vi "EVM_Sweep_Only_R_S_CMP180_DebugMode.vi"() -> ()   [LabVIEW 2023, in "EVM.lvlib"]
uses:
  lib/CTL/LitePoint_EVM_SG.ctl
  lib/CTL/LitePoint_EVM_SA.ctl
  lib/CTL/JIO_FPGA_FTDI.ctl
  EVM.lvlib
  lib/LitePoints/LitePoints.lvlib
  lib/FTDI/JIO/CLC_JIO_FTDI.lvlib
  lib/R_S/R_S.lvlib
panel:
  in  "Init Func.":enum16{"ALL", "BFIC", "UDIC", "OFF"}(ring)
  in  "Recoder?":bool
  out "ReceivedPower":dbl format="%#.3g"
  out "Best EVM ALL":dbl
  out "PST(sec)":dbl
  out "Best EVM":dbl
  out "error out":errorcluster
  in  "Power res":i32=2
  in  "Stop Power":i32
  in  "Start Power":i32=-40
  in  "BFIC_ele_stop":i32=12
  in  "BFIC_ele_res":i32=4
  in  "BFIC_ele_start":i32
  in  "BFIC_com_stop":i32=12
  in  "BFIC_com_res":i32=4
  in  "BFIC_com_start":i32
  in  "UD_att_stop":i32=120
  in  "UD_att_res":i32=8
  in  "UD_att_start":i32
  out "UD_att":i32=255
  out "BFIC_com_step":i32=15
  out "BFIC_ele_step":i32=15
  out "SG Power":i32=-10
  in  "TRXmode":u16(ring)=1 items=["Tx"=1, "Rx"=2]
  in  "Polarity":u16(ring) items=["H", "V"]
  out "floder Exist?":bool=TRUE
  in  "Waiting \nTime(ms)":u32=1
  in  "FileNote":string="test16_wayne_MCS11"
  in  "SG":refnum<visa-resource-name>="TCPIP0::192.168.200.50::hislip0::INSTR"
  in  "SA":refnum<visa-resource-name>="TCPIP0::192.168.200.50::hislip0::INSTR"
  out "Spectrum Data":cluster{"X":dbl, "Y":dbl}[](graph)
  # "TMYTEK_CLC_JIO_R&S_EVM_CMP180_debugMode"
  # "12"
  # "12"
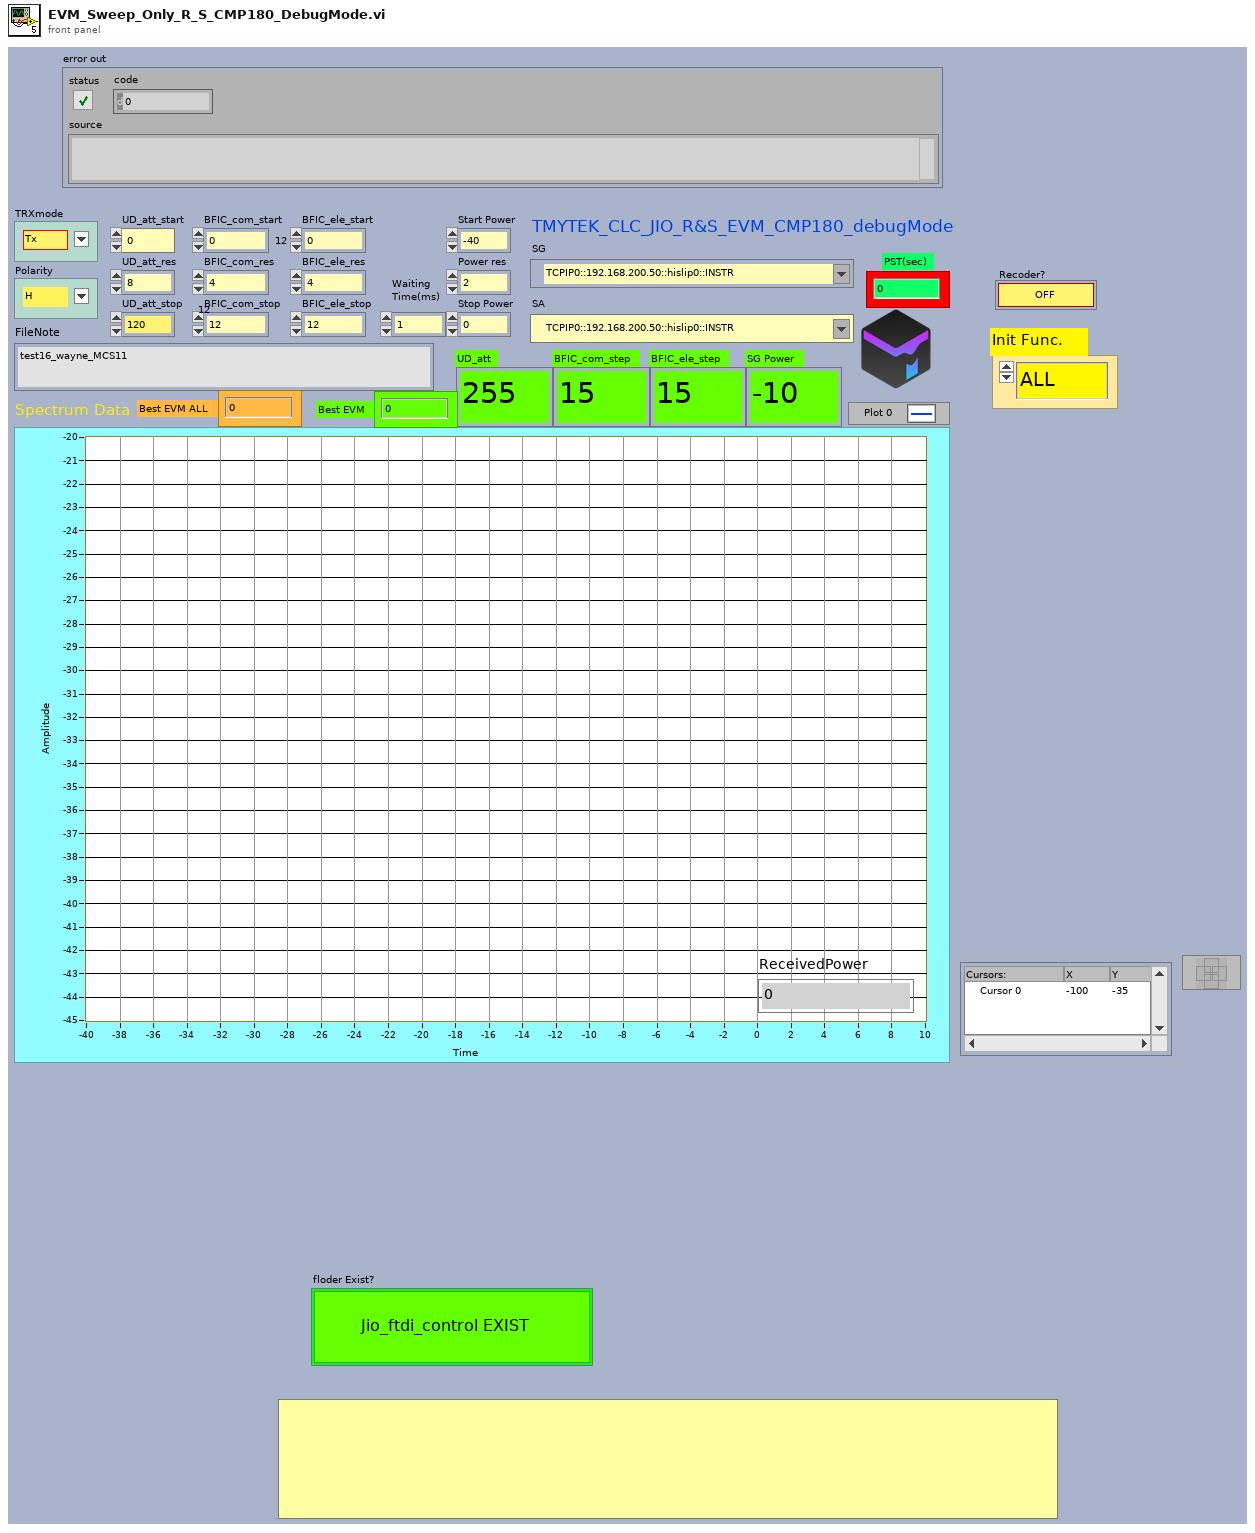
[diagram p1: front panel]
types:
  T1 = typedef "LitePoint_EVM_SG.ctl" = enum16{"Init", "Close", "set_SG", "AdjustLevel", "byPass", "RF_ON", "RF_OFF"}
  T2 = typedef "LitePoint_EVM_SA.ctl" = enum16{"Init", "Close", "set_SA", "get_EVM", "byPass", "getPower"}
  T3 = typedef "JIO_FPGA_FTDI.ctl" = enum16{"Init", "Close", "UD", "BFIC"}
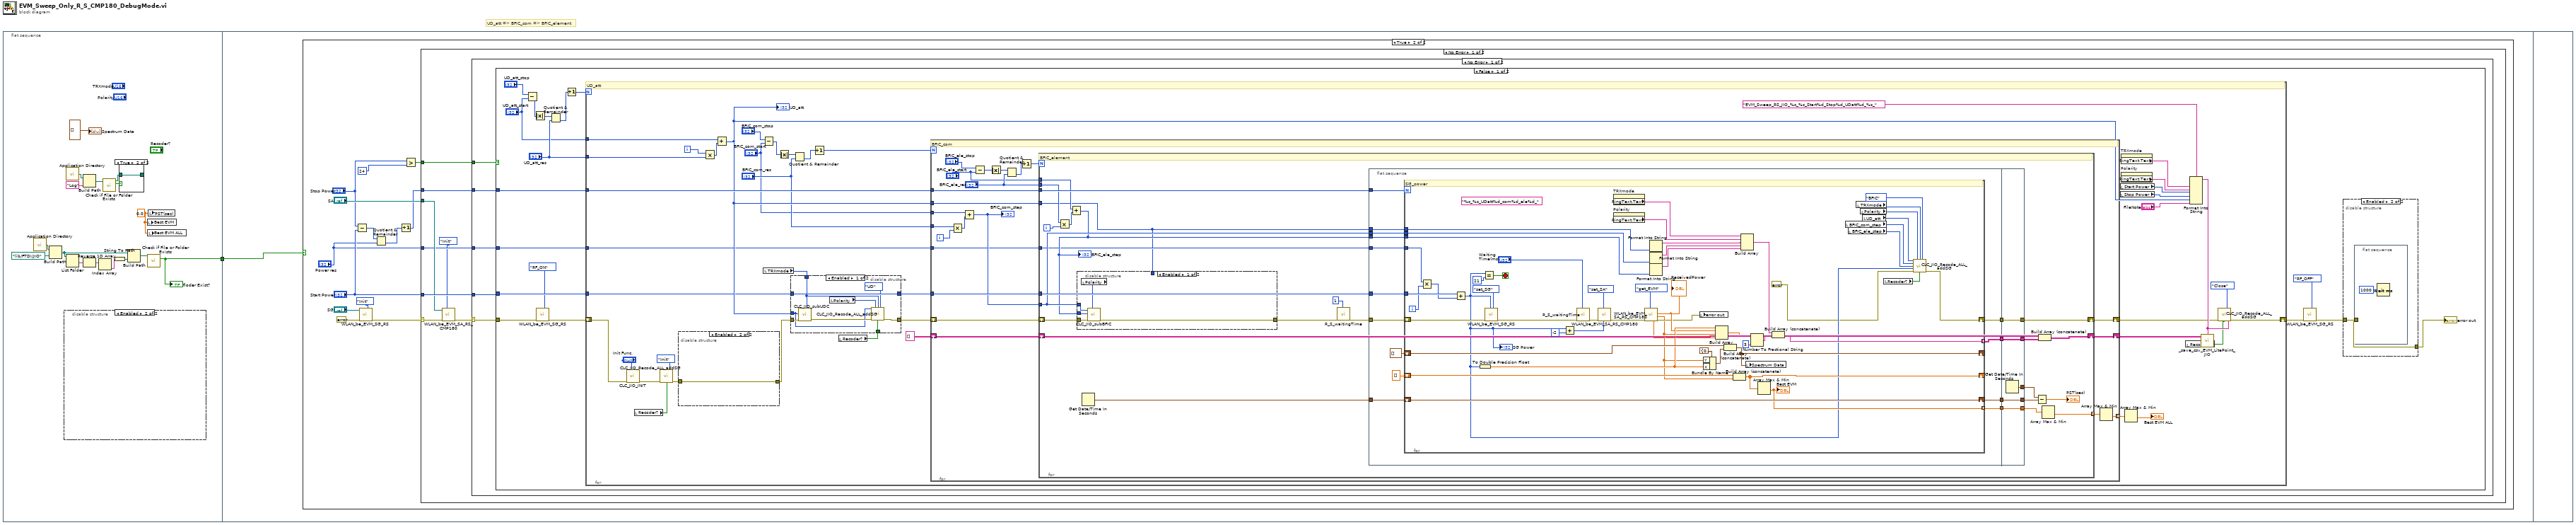
[diagram p0: block diagram]
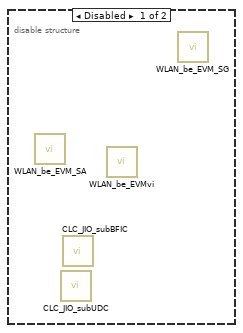
[diagram p2: hidden frame]
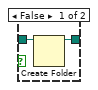
[diagram p3: hidden frame]
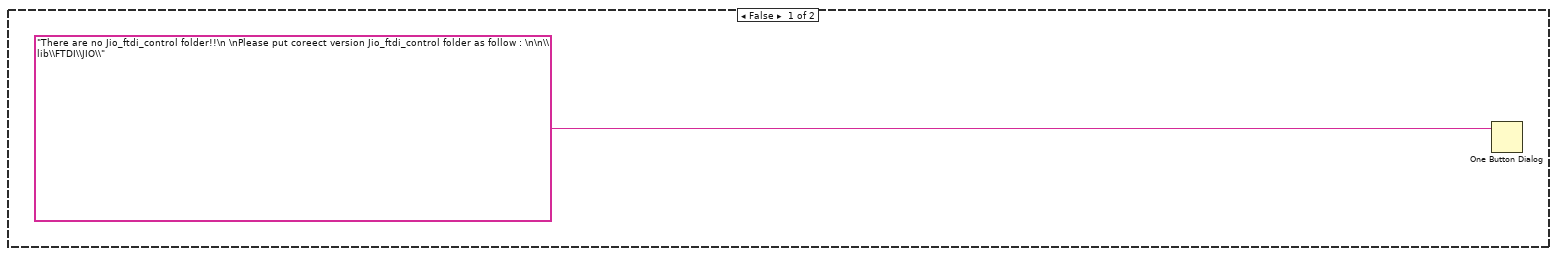
[diagram p4: hidden frame]
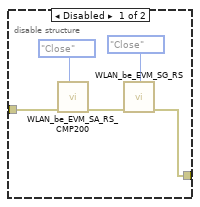
[diagram p5: hidden frame]
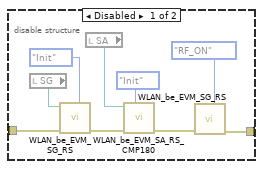
[diagram p6: hidden frame]
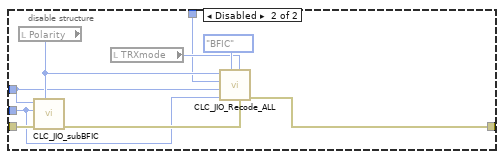
[diagram p8: hidden frame]
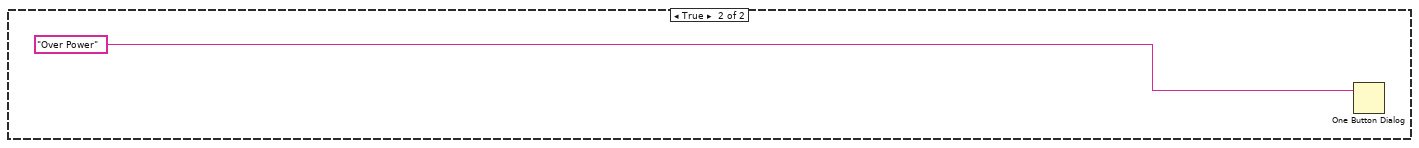
[diagram p9: hidden frame]
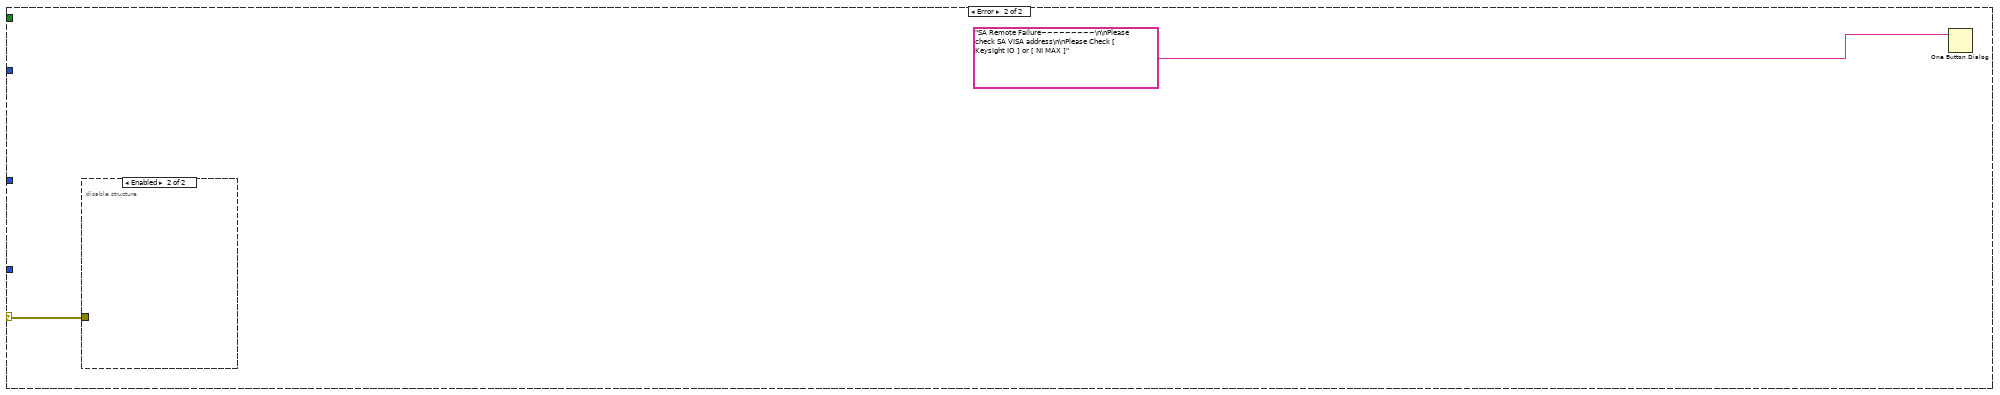
[diagram p10: hidden frame]
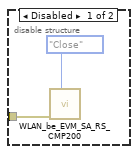
[diagram p11: hidden frame]
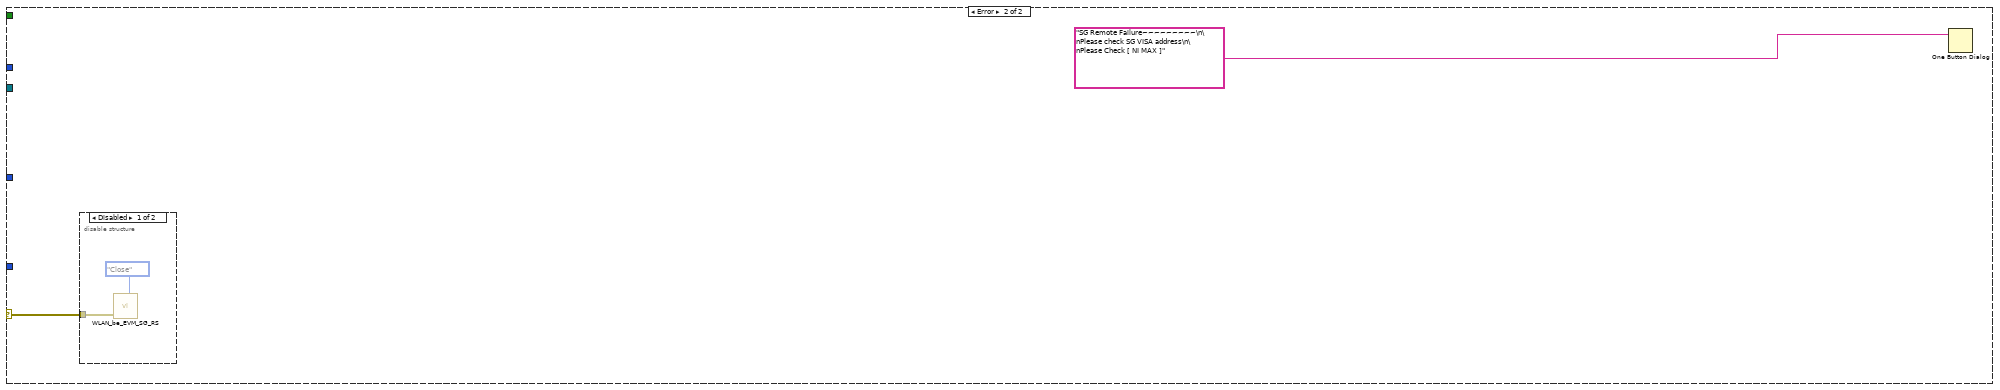
[diagram p12: hidden frame]
diagram:
  # "UD_att => BFIC_com => BFIC_element"
  n1 = flat-sequence {
    tunnel: [w3] -> w1
    tunnel: w1 -> [w21]
    frame #0 {
      w2 = 0.0 ("PST(sec)")
      n2 = call <vilib>:"Application Directory.vi"() -> ("Application Directory"=w9:path)
      n3 = Build Path(base path=w9, name or relative path=path "lib/FTDI/JIO") -> (appended path=w10:path)
      n4 = disable-structure shown="Enabled" {
        frame Disabled {
          n5 = call "WLAN_be_EVM_SA.vi"() -> ()  [unwired: 8 in, 4 out]
          n6 = call "CLC_JIO_subUDC.vi"() -> ()  [unwired: 10 in, 2 out]
          n7 = call "CLC_JIO_subBFIC.vi"() -> ()  [unwired: 10 in, 2 out]
          n8 = call "WLAN_be_EVMvi.vi"() -> ()  [unwired: 8 in, 4 out]
          n9 = call "WLAN_be_EVM_SG.vi"() -> ()  [unwired: 10 in, 2 out]
        }
        frame Enabled {
        }
      }
      n10 = call <vilib>:"Application Directory.vi"() -> ("Application Directory"=w16:path)
      n11 = List Folder(path=w10) -> (folder names=w5:string[])  [unwired: 3 in, 3 out]
      n12 = Reverse 1D Array(array=w5) -> (reversed array=w6:string[])
      n13 = Build Path(base path=w16, name or relative path="Log") -> (appended path=w13:path)
      n14 = Index Array(array=w6) -> (element=w7:string)  [unwired: 1 in]
      n15 = call <vilib>:"Check if File or Folder Exists.vi"("path"=w13) -> ("file or folder exists?"=w15:bool, "dup path"=w14:path)  [unwired: 8 in, 1 out]
      n16 = String To Path(string=w7) -> (path=w8:path)
      n17 = case shown="True" w15 {
        tunnel: w14 -> [w19 w20]
        tunnel: [w18 w20] -> _
        frame False {
          n18 = Create Folder(path (use dialog)=w19) -> (created path=w18:path)  [unwired: 2 in, 2 out]
        }
        frame True {
        }
      }
      n19 = Build Path(base path=w10, name or relative path=w8) -> (appended path=w11:path)
      n20 = local write "Best EVM"(w2) -> ()
      n21 = local write "Best EVM ALL"(w2) -> ()
      n22 = call <vilib>:"Check if File or Folder Exists.vi"("path"=w11) -> ("file or folder exists?"=w3:bool)  [unwired: 8 in, 2 out]
      "floder Exist?" <- w3
      n23 = local write "PST(sec)"(w2) -> ()
      "Spectrum Data" <- cluster{"X":dbl, "Y":dbl}[] [] ("XY Graph")
    }
    frame #1 {
      n24 = case shown="True" w21 {
        frame False {
          n25 = One Button Dialog(message="There are no Jio_ftdi_control folder!!\n \nPlease put coreect version Jio_ftdi_control folder as follow : \n\n\\lib\\FTDI\\JIO\\") -> ()  [unwired: 1 in, 1 out]
        }
        frame True {
          n26 = Subtract(x="Stop Power", y="Start Power") -> (x-y=w26:i32)
          n27 = call "WLAN_be_EVM_SG_RS.vi"("Function_SG"=LitePoint_EVM_SG."Init", "error in"=errorcluster {"status"=FALSE, "code"=0, "source"=""} ("error in (no error)"), "VISA IN"="SG") -> ("error out"=w28:errorcluster)  [unwired: 7 in, 1 out]
          n28 = Quotient & Remainder(x=w26, y="Power res") -> (floor(x/y)=w25:i32)  [unwired: 1 out]
          n29 = Increment(x=w25) -> (x+1=w32:i32)
          n30 = Greater?(x="Stop Power", y=24) -> (0:w34:bool)
          n31 = case shown="No Error" w28 {
            selector: w28 -> [w40 w276]
            tunnel: "SA" -> [w38 _]
            tunnel: w34 -> [w43 _]
            tunnel: "Start Power" -> [w42 _]
            tunnel: w32 -> [w41 _]
            tunnel: "Power res" -> [w37 _]
            frame No Error {
              n32 = call "WLAN_be_EVM_SA_RS_CMP180.vi"("Function"=LitePoint_EVM_SA."Init", "error in"=w40, "VISA IN"=w38) -> ("error out"=w39:errorcluster)  [unwired: 4 in, 4 out]
              n33 = case shown="No Error" w39 {
                selector: w39 -> [w45 w272]
                tunnel: w43 -> [w48 _]
                tunnel: w42 -> [w47 _]
                tunnel: w41 -> [w46 _]
                tunnel: w37 -> [w44 _]
                frame No Error {
                  n34 = case shown="False" w48 {
                    tunnel: w47 -> [w64 _]
                    tunnel: w45 -> [w63 _]
                    tunnel: w46 -> [w65 _]
                    tunnel: w44 -> [w52 _]
                    frame False {
                      n35 = Subtract(x="UD_att_stop", y="UD_att_start") -> (x-y=w59:i32)
                      n36 = Absolute Value(x=w59) -> (abs(x)=w56:i32)
                      n37 = call "WLAN_be_EVM_SG_RS.vi"("Function_SG"=LitePoint_EVM_SG."RF_ON", "error in"=w63) -> ("error out"=w61:errorcluster)  [unwired: 8 in, 1 out]
                      n38 = Quotient & Remainder(x=w56, y="UD_att_res") -> (floor(x/y)=w57:i32)  [unwired: 1 out]
                      n39 = Increment(x=w57) -> (x+1=w53:i32)
                      n40 = for {
                        N: w53 -> [_]
                        tunnel: w65 -> [w115]
                        tunnel: w64 -> [w88]
                        shift-right: [w84] -> w60
                        shift-left: w61 -> [w80]
                        tunnel: "UD_att_res" -> [w102]
                        tunnel: "UD_att_start" -> [w101]
                        tunnel: w52 -> [w92]
                        i -> [w104]
                        # "UD_att"
                        n41 = call "CLC_JIO_INIT.vi"("Func."="Init Func.", "error in"=w80) -> ("error out"=w79:errorcluster)  [unwired: 8 in, 1 out]
                        n42 = local read "Recoder?"() -> (w78:bool)
                        n43 = call "CLC_JIO_Recode_ALL_addSG.vi"("Function"=JIO_FPGA_FTDI."Init", "error in"=w79, "Enable?"=w78) -> ("error out"=w85:errorcluster)  [unwired: 12 in]
                        n44 = disable-structure shown="Enabled" {
                          disable-tunnel: [w122 w125] -> w91
                          disable-tunnel: w85 -> [w121 w125]
                          frame Disabled {
                            n45 = local read "SG"() -> (w117:refnum<visa-resource-name>)
                            n46 = call "WLAN_be_EVM_SG_RS.vi"("Function_SG"=LitePoint_EVM_SG."Init", "error in"=w121, "VISA IN"=w117) -> ("error out"=w118:errorcluster)  [unwired: 7 in, 1 out]
                            n47 = local read "SA"() -> (w116:refnum<visa-resource-name>)
                            n48 = call "WLAN_be_EVM_SA_RS_CMP180.vi"("Function"=LitePoint_EVM_SA."Init", "error in"=w118, "VISA IN"=w116) -> ("error out"=w123:errorcluster)  [unwired: 4 in, 4 out]
                            n49 = call "WLAN_be_EVM_SG_RS.vi"("Function_SG"=LitePoint_EVM_SG."RF_ON", "error in"=w123) -> ("error out"=w122:errorcluster)  [unwired: 8 in, 1 out]
                          }
                          frame Enabled {
                          }
                        }
                        n50 = Multiply(x=w104, y=w102) -> (x*y=w103:i32)
                        n51 = Add(x=w101, y=w103) -> (x+y=w100:i32)
                        "UD_att" <- w100
                        n52 = Subtract(x="BFIC_com_stop", y="BFIC_com_start") -> (x-y=w99:i32)
                        n53 = local read "TRXmode"() -> (w112:u16)
                        n54 = Absolute Value(x=w99) -> (abs(x)=w98:i32)
                        n55 = Quotient & Remainder(x=w98, y="BFIC_com_res") -> (floor(x/y)=w94:i32)  [unwired: 1 out]
                        n56 = Increment(x=w94) -> (x+1=w93:i32)
                        n57 = local read "Recoder?"() -> (w77:bool)
                        n58 = disable-structure shown="Enabled" {
                          disable-tunnel: [w132 w135] -> w114
                          disable-tunnel: w91 -> [w134 w135]
                          disable-tunnel: w112 -> [w129 _]
                          disable-tunnel: w100 -> [w128 _]
                          disable-tunnel: [w131 _] -> w87
                          disable-tunnel: w88 -> [w131 _]
                          disable-tunnel: w77 -> [w126 _]
                          frame Enabled {
                            n59 = call "CLC_JIO_subUDC.vi"("Mode"=w129, "error in"=w134, "ud att"=w128) -> ("error out"=w133:errorcluster)  [unwired: 7 in, 1 out]
                            n60 = local read "Polarity"() -> (w127:u16)
                            n61 = call "CLC_JIO_Recode_ALL_addSG.vi"("UD_att"=w128, "pol"=w127, "Mode"=w129, "Function"=JIO_FPGA_FTDI."UD", "error in"=w133, "Enable?"=w126) -> ("error out"=w132:errorcluster)  [unwired: 9 in]
                          }
                          frame Disabled {
                          }
                        }
                        n62 = for {
                          N: w93 -> [_]
                          tunnel: w115 -> [w157]
                          tunnel: w87 -> [w156]
                          shift-right: [w153] -> w113
                          shift-left: string[][] [] -> [w154]
                          tunnel: w100 -> [w152]
                          shift-right: [w151] -> w81
                          shift-left: w114 -> [w155]
                          tunnel: "BFIC_com_res" -> [w147]
                          tunnel: "BFIC_com_start" -> [w146]
                          tunnel: w92 -> [w138]
                          tunnel: [w136] -> w90 mode=indexing
                          i -> [w149]
                          # "BFIC_com"
                          n63 = Multiply(x=w147, y=w149) -> (x*y=w150:i32)
                          n64 = Add(x=w146, y=w150) -> (x+y=w148:i32)
                          "BFIC_com_step" <- w148
                          n65 = Subtract(x="BFIC_ele_stop", y="BFIC_ele_start") -> (x-y=w144:i32)
                          n66 = Absolute Value(x=w144) -> (abs(x)=w145:i32)
                          n67 = Quotient & Remainder(x=w145, y="BFIC_ele_res") -> (floor(x/y)=w142:i32)  [unwired: 1 out]
                          n68 = Increment(x=w142) -> (x+1=w139:i32)
                          n69 = for {
                            N: w139 -> [_]
                            tunnel: w157 -> [w185]
                            tunnel: w156 -> [w184]
                            shift-right: [w182] -> w153
                            shift-left: w154 -> [w181]
                            tunnel: w148 -> [w177]
                            tunnel: w152 -> [w158]
                            shift-right: [w162] -> w151
                            shift-left: w155 -> [w180]
                            tunnel: "BFIC_ele_res" -> [w173]
                            tunnel: "BFIC_ele_start" -> [w172]
                            tunnel: w138 -> [w171]
                            tunnel: [w159] -> w137 mode=indexing
                            i -> [w174]
                            # "BFIC_element"
                            n70 = Multiply(x=w173, y=w174) -> (x*y=w176:i32)
                            n71 = Add(x=w172, y=w176) -> (x+y=w175:i32)
                            "BFIC_ele_step" <- w175
                            n72 = disable-structure shown="Enabled" {
                              disable-tunnel: w180 -> [w261 w270]
                              disable-tunnel: [w257 w268] -> w179
                              disable-tunnel: w175 -> [w258 w262]
                              disable-tunnel: w177 -> [w259 w263]
                              disable-tunnel: w158 -> [_ w264]
                              frame Enabled {
                                n73 = local read "Polarity"() -> (w260:u16)
                                n74 = call "CLC_JIO_subBFIC.vi"("pol"=w260, "error in"=w261, "ele"=w258, "com"=w259) -> ("error out"=w257:errorcluster)  [unwired: 6 in, 1 out]
                              }
                              frame Disabled {
                                n75 = local read "Polarity"() -> (w265:u16)
                                n76 = call "CLC_JIO_subBFIC.vi"("pol"=w265, "error in"=w270, "ele"=w262, "com"=w263) -> ("error out"=w269:errorcluster)  [unwired: 6 in, 1 out]
                                n77 = local read "TRXmode"() -> (w266:u16)
                                n78 = call "CLC_JIO_Recode_ALL.vi"("error in"=w269, "Mode"=w266, "Function"=JIO_FPGA_FTDI."BFIC", "ele_att"=w262, "com_att"=w263, "UD_att"=w264, "pol"=w265) -> ("error out"=w268:errorcluster)  [unwired: 3 in, 1 out]
                              }
                            }
                            n79 = Get Date/Time In Seconds() -> (seconds since 1Jan1904=w169:timestamp)
                            n80 = call "R_S_waitingTime.vi"("Waiting Time(ms)"=u32 1, "error in"=w179) -> ("error out"=w170:errorcluster)  [unwired: 9 in]
                            n81 = flat-sequence {
                              tunnel: w185 -> [w199]
                              tunnel: w184 -> [w197]
                              tunnel: w158 -> [w195]
                              tunnel: w177 -> [w194]
                              tunnel: w175 -> [w192]
                              tunnel: w171 -> [w191]
                              tunnel: w170 -> [w190]
                              tunnel: w169 -> [w188]
                              tunnel: [w196] -> w167
                              tunnel: [w193] -> w166
                              tunnel: [w187] -> w165
                              tunnel: [w186] -> w161
                              tunnel: w167 -> [w256]
                              tunnel: w166 -> [w255]
                              tunnel: w165 -> [w254]
                              tunnel: w161 -> [w252]
                              tunnel: [w256] -> w183
                              tunnel: [w255] -> w162
                              tunnel: [w254] -> w168
                              tunnel: [w253] -> w164
                              tunnel: [w252] -> w160
                              frame #0 {
                                n82 = for {
                                N: w199 -> [_]
                                tunnel: w197 -> [w251]
                                shift-right: [w201] -> w193
                                shift-left: w190 -> [w243]
                                shift-right: [w245] -> _
                                shift-left: cluster{"X":dbl, "Y":dbl}[] [] ("XY Graph") -> [w247]
                                tunnel: [w235] -> w196 mode=indexing
                                tunnel: w195 -> [w232]
                                tunnel: w192 -> [w230]
                                tunnel: w194 -> [w231]
                                tunnel: w191 -> [w224]
                                shift-right: [w213] -> _
                                shift-left: dbl[] [] -> [w215]
                                shift-right: [w212] -> w187
                                shift-left: w188 -> [w212]
                                tunnel: [w211] -> w186 mode=indexing
                                i -> [w225]
                                stop <- w249 stop-if-true
                                (unwired) "%s_%s_UDatt%d_com%d_ele%d_" ("format string")
                                # "SG_power"
                                n83 = Multiply(x=w224, y=w225) -> (x*y=w223:i32)
                                n84 = Add(x=w251, y=w223) -> (x+y=w203:i32)
                                "SG Power" <- w203
                                n85 = To Double Precision Float(number=w203) -> (double precision float=w244:dbl)
                                n86 = Equal?(x=w203, y=21) -> (x = y?=w249:bool)
                                n87 = call "WLAN_be_EVM_SG_RS.vi"("Function_SG"=LitePoint_EVM_SG."set_SG", "setPower"=w203, "error in"=w243) -> ("error out"=w221:errorcluster)  [unwired: 7 in, 1 out]
                                n88 = Add(x=w203, y=-2) -> (x+y=w217:i32)
                                n89 = call "R_S_waitingTime.vi"("Waiting Time(ms)"="Waiting \nTime(ms)", "error in"=w221) -> ("error out"=w239:errorcluster)  [unwired: 9 in]
                                n90 = call "WLAN_be_EVM_SA_RS_CMP180.vi"("SG Power"=w217, "Function"=LitePoint_EVM_SA."set_SA", "error in"=w239) -> ("error out"=w219:errorcluster)  [unwired: 4 in, 4 out]
                                n91 = property on="TRXmode" class="Ring (strict)"() -> ("RingText.Text"=w234:string)  [unwired: 2 in, 2 out]
                                n92 = property on="Polarity" class="Ring (strict)"() -> ("RingText.Text"=w233:string)  [unwired: 2 in, 2 out]
                                n93 = call "WLAN_be_EVM_SA_RS_CMP180.vi"("Function"=LitePoint_EVM_SA."get_EVM", "error in"=w219) -> ("error out"=w218:errorcluster, "EVM"=w214:dbl, "Power"=w222:dbl, "FreqError"=w210:dbl)  [unwired: 5 in, 1 out]
                                "ReceivedPower" <- w222
                                n94 = Format Into String(w232) -> (resulting string=w229:string)  [unwired: 3 in, 1 out]
                                n95 = Format Into String(w231) -> (resulting string=w228:string)  [unwired: 3 in, 1 out]
                                n96 = Format Into String(w230) -> (resulting string=w227:string)  [unwired: 3 in, 1 out]
                                n97 = local write "error out"(w218) -> ()
                                n98 = Bundle By Name(cluster=cluster{"X":dbl, "Y":dbl} {"X"=0.0, "Y"=0.0} ("element"), "Y"=w214, "X"=w244) -> (w246:cluster{"X":dbl, "Y":dbl})
                                n99 = Build Array(w244, w222, w214, w210) -> (w237:dbl[])
                                n100 = Build Array (concatenate)(w247, w246) -> (w245:cluster{"X":dbl, "Y":dbl}[])
                                n101 = Build Array (concatenate)(w215, w214) -> (w213:dbl[])
                                n102 = Build Array(w234, w233, w229, w228, w227) -> (w226:string[])
                                n103 = local write "Spectrum Data"(w245) -> ()
                                n104 = Number To Fractional String(number=w237, precision (6)=i16 3) -> (F-format string=w236:string[])  [unwired: 2 in]
                                n105 = Array Max & Min(array=w213) -> (min value=w211:dbl)  [unwired: 3 out]
                                "Best EVM" <- w211
                                n106 = Build Array (concatenate)(w226, w236) -> (w235:string[])
                                n107 = local read "BFIC_com_step"() -> (w205:i32)
                                n108 = local read "BFIC_ele_step"() -> (w204:i32)
                                n109 = local read "TRXmode"() -> (w208:u16)
                                n110 = local read "Polarity"() -> (w207:u16)
                                n111 = local read "UD_att"() -> (w206:i32)
                                n112 = local read "Recoder?"() -> (w200:bool)
                                n113 = call "CLC_JIO_Recode_ALL_addSG.vi"("UD_att"=w206, "pol"=w207, "Mode"=w208, "Function"=JIO_FPGA_FTDI."BFIC", "com_att"=w205, "ele_att"=w204, "SG Power"=w203, "error in"=errorcluster {"status"=FALSE, "code"=0, "source"=""} ("error out"), "Enable?"=w200) -> ("error out"=w201:errorcluster)  [unwired: 6 in]
                                }
                              }
                              frame #1 {
                                n114 = Get Date/Time In Seconds() -> (seconds since 1Jan1904=w253:timestamp)
                              }
                            }
                            n115 = Subtract(x=w164, y=w168) -> (x-y=→"PST(sec)":dbl)
                            n116 = Build Array (concatenate)(w181, w183) -> (w182:string[][])
                            n117 = Array Max & Min(array=w160) -> (min value=w159:dbl)  [unwired: 3 out]
                          }
                          n118 = Array Max & Min(array=w137) -> (min value=w136:dbl)  [unwired: 3 out]
                        }
                        n119 = local read "Start Power"() -> (w108:i32)
                        n120 = local read "Stop Power"() -> (w110:i32)
                        n121 = property on="TRXmode" class="Ring (strict)"() -> ("RingText.Text"=w106:string)  [unwired: 2 in, 2 out]
                        n122 = property on="Polarity" class="Ring (strict)"() -> ("RingText.Text"=w107:string)  [unwired: 2 in, 2 out]
                        n123 = Array Max & Min(array=w90) -> (min value=→"Best EVM ALL":dbl)  [unwired: 3 out]
                        n124 = local read "Recoder?"() -> (w76:bool)
                        n125 = Format Into String(format string="EVM_Sweep_RS_JIO_%s_%s_Start%d_Stop%d_UDatt%d_%s_" ("delimiter (\\t)"), w106, w107, w108, w110, w100, "FileNote") -> (resulting string=w82:string)  [unwired: 2 in, 1 out]
                        n126 = call "_save_csv_EVM_LitePoint_JIO.vi"("delimiter (\\t)"=w82, "array in"=w113) -> ()  [unwired: 9 in, 1 out]
                        n127 = call "CLC_JIO_Recode_ALL_addSG.vi"("Function"=JIO_FPGA_FTDI."Close", "error in"=w81, "Enable?"=w76, "FileName"=w82) -> ("error out"=w84:errorcluster)  [unwired: 11 in]
                      }
                      n128 = call "WLAN_be_EVM_SG_RS.vi"("Function_SG"=LitePoint_EVM_SG."RF_OFF", "error in"=w60) -> ("error out"=w50:errorcluster)  [unwired: 8 in, 1 out]
                      n129 = disable-structure shown="Enabled" {
                        disable-tunnel: w50 -> [w69 w72]
                        disable-tunnel: [w66 w71] -> w49
                        frame Disabled {
                          n130 = call "WLAN_be_EVM_SA_RS_CMP200.vi"("Function"=LitePoint_EVM_SA."Close", "error in"=w69) -> ("error out"=w68:errorcluster)  [unwired: 6 in, 3 out]
                          n131 = call "WLAN_be_EVM_SG_RS.vi"("Function_SG"=LitePoint_EVM_SG."Close", "error in"=w68) -> ("error out"=w66:errorcluster)  [unwired: 8 in, 1 out]
                        }
                        frame Enabled {
                          n132 = flat-sequence {
                            tunnel: [w74] -> w71
                            tunnel: w72 -> [w74]
                            frame #0 {
                              n133 = Wait (ms)(milliseconds to wait=u32 1000) -> ()  [unwired: 1 out]
                            }
                          }
                        }
                      }
                      "error out" <- w49
                    }
                    frame True {
                      n134 = One Button Dialog(message="Over Power") -> ()  [unwired: 1 in, 1 out]
                    }
                  }
                }
                frame Error {
                  n135 = disable-structure shown="Enabled" {
                    disable-tunnel: w272 -> [w275 _]
                    frame Disabled {
                      n136 = call "WLAN_be_EVM_SA_RS_CMP200.vi"("Function"=LitePoint_EVM_SA."Close", "error in"=w275) -> ()  [unwired: 6 in, 4 out]
                    }
                    frame Enabled {
                    }
                  }
                  n137 = One Button Dialog(message="SA Remote Failure~~~~~~~~~\n\nPlease check SA VISA address\n\nPlease Check [ Keysight IO ] or [ NI MAX ]") -> ()  [unwired: 1 in, 1 out]
                }
              }
            }
            frame Error {
              n138 = disable-structure shown="Disabled" {
                disable-tunnel: w276 -> [w279 _]
                frame Disabled {
                  n139 = call "WLAN_be_EVM_SG_RS.vi"("Function_SG"=LitePoint_EVM_SG."Close", "error in"=w279) -> ()  [unwired: 8 in, 2 out]
                }
                frame Enabled {
                }
              }
              n140 = One Button Dialog(message="SG Remote Failure~~~~~~~~~\n\nPlease check SG VISA address\n\nPlease Check [ NI MAX ]") -> ()  [unwired: 1 in, 1 out]
            }
          }
        }
      }
    }
    frame #2 {
    }
  }
